vi "Create Stream Writer.vi"(8 "error in (no error)":errorcluster, 11 "Shell Stream Ref":refnum<k24>) -> (0 "error out":errorcluster, 2 "Stream Writer ref":refnum<k24>)   [LabVIEW 2017, in "SSH.lvlib"]
uses:
  SSH.lvlib
  C:/Users/phorn/Documents/LV_SSH/Renci.SshNet.dll
  Renci.SshNet.dll
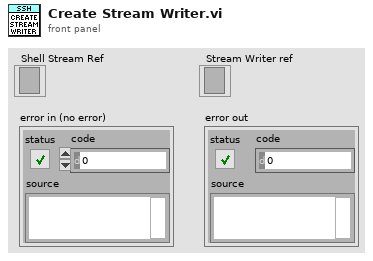
[diagram p1: front panel]
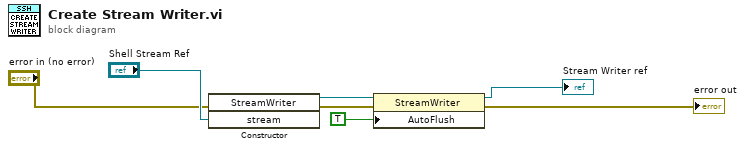
[diagram p0: block diagram]
diagram:
  n1 = constructor class="StreamWriter"(error in="error in (no error)", "stream"="Shell Stream Ref") -> (reference out=w3:refnum<k24>, error out=w2:errorcluster)  [unwired: 2 in, 2 out]
  n2 = property class="StreamWriter"(reference=w3, error in=w2, "AutoFlush"=TRUE) -> (reference out=→"Stream Writer ref":refnum<k24>, error out=→"error out":errorcluster)
